vi "Create PMUs.vi"(8 "error in (no error)":errorcluster) -> (0 "error out":errorcluster)   [LabVIEW 2013, in "PMU Recorder Light.lvlib" / "Phasor Measurement Unit.lvclass"]
uses:
  Phasor Measurement Unit.lvclass
panel:
  in  "PMU Configuration":T1
  in  "Test Configuration":T1={"PMU Configuration"=[{"PMU ID Code"=3, "Station Name"="Hasle           ", "Nominal Frequency"=50.0, "Format Code"=8, "Configuration Change Count"=0, "Number of Phasors"=6, "Number of Analog"=0, "Number of Digital"=0, "Status"=TRUE}, {"PMU ID Code"=0, "Station Name"="NedreRossaga    ", "Nominal Frequency"=50.0, "Format Code"=8, "Configuration Change Count"=1, "Number of Phasors"=2, "Number of Analog"=0, "Number of Digital"=0, "Status"=TRUE}, {"PMU ID Code"=0, "Station Name"="Ben 667         ", "Nominal Frequency"=50.0, "Format Code"=8, "Configuration Change Count"=1, "Number of Phasors"=12, "Number of Analog"=0, "Number of Digital"=0, "Status"=TRUE}, {"PMU ID Code"=102, "Station Name"="Keminmaa        ", "Nominal Frequency"=50.0, "Format Code"=8, "Configuration Change Count"=4, "Number of Phasors"=6, "Number of Analog"=0, "Number of Digital"=0, "Status"=TRUE}, {"PMU ID Code"=113, "Station Name"="PETAJASKOSKI    ", "Nominal Frequency"=50.0, "Format Code"=8, "Configuration Change Count"=9, "Number of Phasors"=3, "Number of Analog"=0, "Number of Digital"=0, "Status"=TRUE}], "Phasor Configuration"=[{"Group Name"="Hasle", "Channel Name"="Halden-U", "Channel Name Real"="Halden-U", "Channel Name Imaginary"="Halden-U", "Group Index"=0, "Channel Index"=0, "isValid?"=TRUE, "Scaling"=20.97388, "Type"=0}, {"Group Name"="Hasle", "Channel Name"="Borgvik-U", "Channel Name Real"="Borgvik-U", "Channel Name Imaginary"="Borgvik-U", "Group Index"=0, "Channel Index"=1, "isValid?"=TRUE, "Scaling"=20.97388, "Type"=0}, {"Group Name"="Hasle", "Channel Name"="Borgvik-I", "Channel Name Real"="Borgvik-I", "Channel Name Imaginary"="Borgvik-I", "Group Index"=0, "Channel Index"=2, "isValid?"=TRUE, "Scaling"=0.54931, "Type"=1}, {"Group Name"="Hasle", "Channel Name"="Halden-I", "Channel Name Real"="Halden-I", "Channel Name Imaginary"="Halden-I", "Group Index"=0, "Channel Index"=3, "isValid?"=TRUE, "Scaling"=0.54931, "Type"=1}, {"Group Name"="Hasle", "Channel Name"="Roed-I", "Channel Name Real"="Roed-I", "Channel Name Imaginary"="Roed-I", "Group Index"=0, "Channel Index"=4, "isValid?"=TRUE, "Scaling"=0.54931, "Type"=1}, {"Group Name"="Hasle", "Channel Name"="Tegneby-I", "Channel Name Real"="Tegneby-I", "Channel Name Imaginary"="Tegneby-I", "Group Index"=0, "Channel Index"=5, "isValid?"=TRUE, "Scaling"=0.73242, "Type"=1}, {"Group Name"="NedreRossaga", "Channel Name"="Rana-U", "Channel Name Real"="Rana-U", "Channel Name Imaginary"="Rana-U", "Group Index"=1, "Channel Index"=0, "isValid?"=TRUE, "Scaling"=19.97513, "Type"=0}, {"Group Name"="NedreRossaga", "Channel Name"="Rana-I", "Channel Name Real"="Rana-I", "Channel Name Imaginary"="Rana-I", "Group Index"=1, "Channel Index"=1, "isValid?"=TRUE, "Scaling"=0.05493, "Type"=1}, {"Group Name"="Ben 667", "Channel Name"="420:Ba1:U_L1", "Channel Name Real"="420:Ba1:U_L1", "Channel Name Imaginary"="420:Ba1:U_L1", "Group Index"=2, "Channel Index"=0, "isValid?"=TRUE, "Scaling"=14.76031, "Type"=0}, {"Group Name"="Ben 667", "Channel Name"="420:Ba1:U_L2", "Channel Name Real"="420:Ba1:U_L2", "Channel Name Imaginary"="420:Ba1:U_L2", "Group Index"=2, "Channel Index"=1, "isValid?"=TRUE, "Scaling"=14.76031, "Type"=0}, {"Group Name"="Ben 667", "Channel Name"="420:Ba1:U_L3", "Channel Name Real"="420:Ba1:U_L3", "Channel Name Imaginary"="420:Ba1:U_L3", "Group Index"=2, "Channel Index"=2, "isValid?"=TRUE, "Scaling"=14.76031, "Type"=0}, {"Group Name"="Ben 667", "Channel Name"="420:Ba1:I_L1", "Channel Name Real"="420:Ba1:I_L1", "Channel Name Imaginary"="420:Ba1:I_L1", "Group Index"=2, "Channel Index"=3, "isValid?"=TRUE, "Scaling"=0.31169, "Type"=1}, {"Group Name"="Ben 667", "Channel Name"="420:Ba1:I_L2", "Channel Name Real"="420:Ba1:I_L2", "Channel Name Imaginary"="420:Ba1:I_L2", "Group Index"=2, "Channel Index"=4, "isValid?"=TRUE, "Scaling"=0.31169, "Type"=1}, {"Group Name"="Ben 667", "Channel Name"="420:Ba1:I_L3", "Channel Name Real"="420:Ba1:I_L3", "Channel Name Imaginary"="420:Ba1:I_L3", "Group Index"=2, "Channel Index"=5, "isValid?"=TRUE, "Scaling"=0.31169, "Type"=1}, {"Group Name"="Ben 667", "Channel Name"="420:Of1:U_L1", "Channel Name Real"="420:Of1:U_L1", "Channel Name Imaginary"="420:Of1:U_L1", "Group Index"=2, "Channel Index"=6, "isValid?"=TRUE, "Scaling"=14.76031, "Type"=0}, {"Group Name"="Ben 667", "Channel Name"="420:Of1:U_L2", "Channel Name Real"="420:Of1:U_L2", "Channel Name Imaginary"="420:Of1:U_L2", "Group Index"=2, "Channel Index"=7, "isValid?"=TRUE, "Scaling"=14.76031, "Type"=0}, {"Group Name"="Ben 667", "Channel Name"="420:Of1:U_L3", "Channel Name Real"="420:Of1:U_L3", "Channel Name Imaginary"="420:Of1:U_L3", "Group Index"=2, "Channel Index"=8, "isValid?"=TRUE, "Scaling"=14.76031, "Type"=0}, {"Group Name"="Ben 667", "Channel Name"="420:Of1:I_L1", "Channel Name Real"="420:Of1:I_L1", "Channel Name Imaginary"="420:Of1:I_L1", "Group Index"=2, "Channel Index"=9, "isValid?"=TRUE, "Scaling"=0.31169, "Type"=1}, {"Group Name"="Ben 667", "Channel Name"="420:Of1:I_L2", "Channel Name Real"="420:Of1:I_L2", "Channel Name Imaginary"="420:Of1:I_L2", "Group Index"=2, "Channel Index"=10, "isValid?"=TRUE, "Scaling"=0.31169, "Type"=1}, {"Group Name"="Ben 667", "Channel Name"="420:Of1:I_L3", "Channel Name Real"="420:Of1:I_L3", "Channel Name Imaginary"="420:Of1:I_L3", "Group Index"=2, "Channel Index"=11, "isValid?"=TRUE, "Scaling"=0.31169, "Type"=1}, {"Group Name"="Keminmaa", "Channel Name"="PK1", "Channel Name Real"="PK1", "Channel Name Imaginary"="PK1", "Group Index"=3, "Channel Index"=0, "isValid?"=TRUE, "Scaling"=21.97265, "Type"=0}, {"Group Name"="Keminmaa", "Channel Name"="PK2", "Channel Name Real"="PK2", "Channel Name Imaginary"="PK2", "Group Index"=3, "Channel Index"=1, "isValid?"=TRUE, "Scaling"=21.97265, "Type"=0}, {"Group Name"="Keminmaa", "Channel Name"="SELLEE 1.1/2", "Channel Name Real"="SELLEE 1.1/2", "Channel Name Imaginary"="SELLEE 1.1/2", "Group Index"=3, "Channel Index"=2, "isValid?"=TRUE, "Scaling"=0.27465, "Type"=1}, {"Group Name"="Keminmaa", "Channel Name"="SB 1.7/8", "Channel Name Real"="SB 1.7/8", "Channel Name Imaginary"="SB 1.7/8", "Group Index"=3, "Channel Index"=3, "isValid?"=TRUE, "Scaling"=0.54931, "Type"=1}, {"Group Name"="Keminmaa", "Channel Name"="PR 1.9/10", "Channel Name Real"="PR 1.9/10", "Channel Name Imaginary"="PR 1.9/10", "Group Index"=3, "Channel Index"=4, "isValid?"=TRUE, "Scaling"=0.27465, "Type"=1}, {"Group Name"="Keminmaa", "Channel Name"="PT 1.11/12", "Channel Name Real"="PT 1.11/12", "Channel Name Imaginary"="PT 1.11/12", "Group Index"=3, "Channel Index"=5, "isValid?"=TRUE, "Scaling"=0.54931, "Type"=1}, {"Group Name"="PETAJASKOSKI", "Channel Name"="V1LPM", "Channel Name Real"="V1LPM", "Channel Name Imaginary"="V1LPM", "Group Index"=4, "Channel Index"=0, "isValid?"=TRUE, "Scaling"=18.31055, "Type"=0}, {"Group Name"="PETAJASKOSKI", "Channel Name"="I1WPM", "Channel Name Real"="I1WPM", "Channel Name Imaginary"="I1WPM", "Group Index"=4, "Channel Index"=1, "isValid?"=TRUE, "Scaling"=0.32043, "Type"=1}, {"Group Name"="PETAJASKOSKI", "Channel Name"="I1XPM", "Channel Name Real"="I1XPM", "Channel Name Imaginary"="I1XPM", "Group Index"=4, "Channel Index"=2, "isValid?"=TRUE, "Scaling"=0.64087, "Type"=1}], "Analog Configuration"=[{"Group Name"="Hasle", "Channel Name"="frequency", "Group Index"=0, "Channel Index"=0, "isValid?"=TRUE, "Scaling"=1.0, "Type"=100}, {"Group Name"="Hasle", "Channel Name"="frequency-delta", "Group Index"=0, "Channel Index"=1, "isValid?"=TRUE, "Scaling"=1.0, "Type"=101}, {"Group Name"="NedreRossaga", "Channel Name"="frequency", "Group Index"=1, "Channel Index"=0, "isValid?"=TRUE, "Scaling"=1.0, "Type"=100}, {"Group Name"="NedreRossaga", "Channel Name"="frequency-delta", "Group Index"=1, "Channel Index"=1, "isValid?"=TRUE, "Scaling"=1.0, "Type"=101}, {"Group Name"="Ben 667", "Channel Name"="frequency", "Group Index"=2, "Channel Index"=0, "isValid?"=TRUE, "Scaling"=1.0, "Type"=100}, {"Group Name"="Ben 667", "Channel Name"="frequency-delta", "Group Index"=2, "Channel Index"=1, "isValid?"=TRUE, "Scaling"=1.0, "Type"=101}, {"Group Name"="Keminmaa", "Channel Name"="frequency", "Group Index"=3, "Channel Index"=0, "isValid?"=TRUE, "Scaling"=1.0, "Type"=100}, {"Group Name"="Keminmaa", "Channel Name"="frequency-delta", "Group Index"=3, "Channel Index"=1, "isValid?"=TRUE, "Scaling"=1.0, "Type"=101}, {"Group Name"="PETAJASKOSKI", "Channel Name"="frequency", "Group Index"=4, "Channel Index"=0, "isValid?"=TRUE, "Scaling"=1.0, "Type"=100}, {"Group Name"="PETAJASKOSKI", "Channel Name"="frequency-delta", "Group Index"=4, "Channel Index"=1, "isValid?"=TRUE, "Scaling"=1.0, "Type"=101}], "Digital Configuration"=[]}
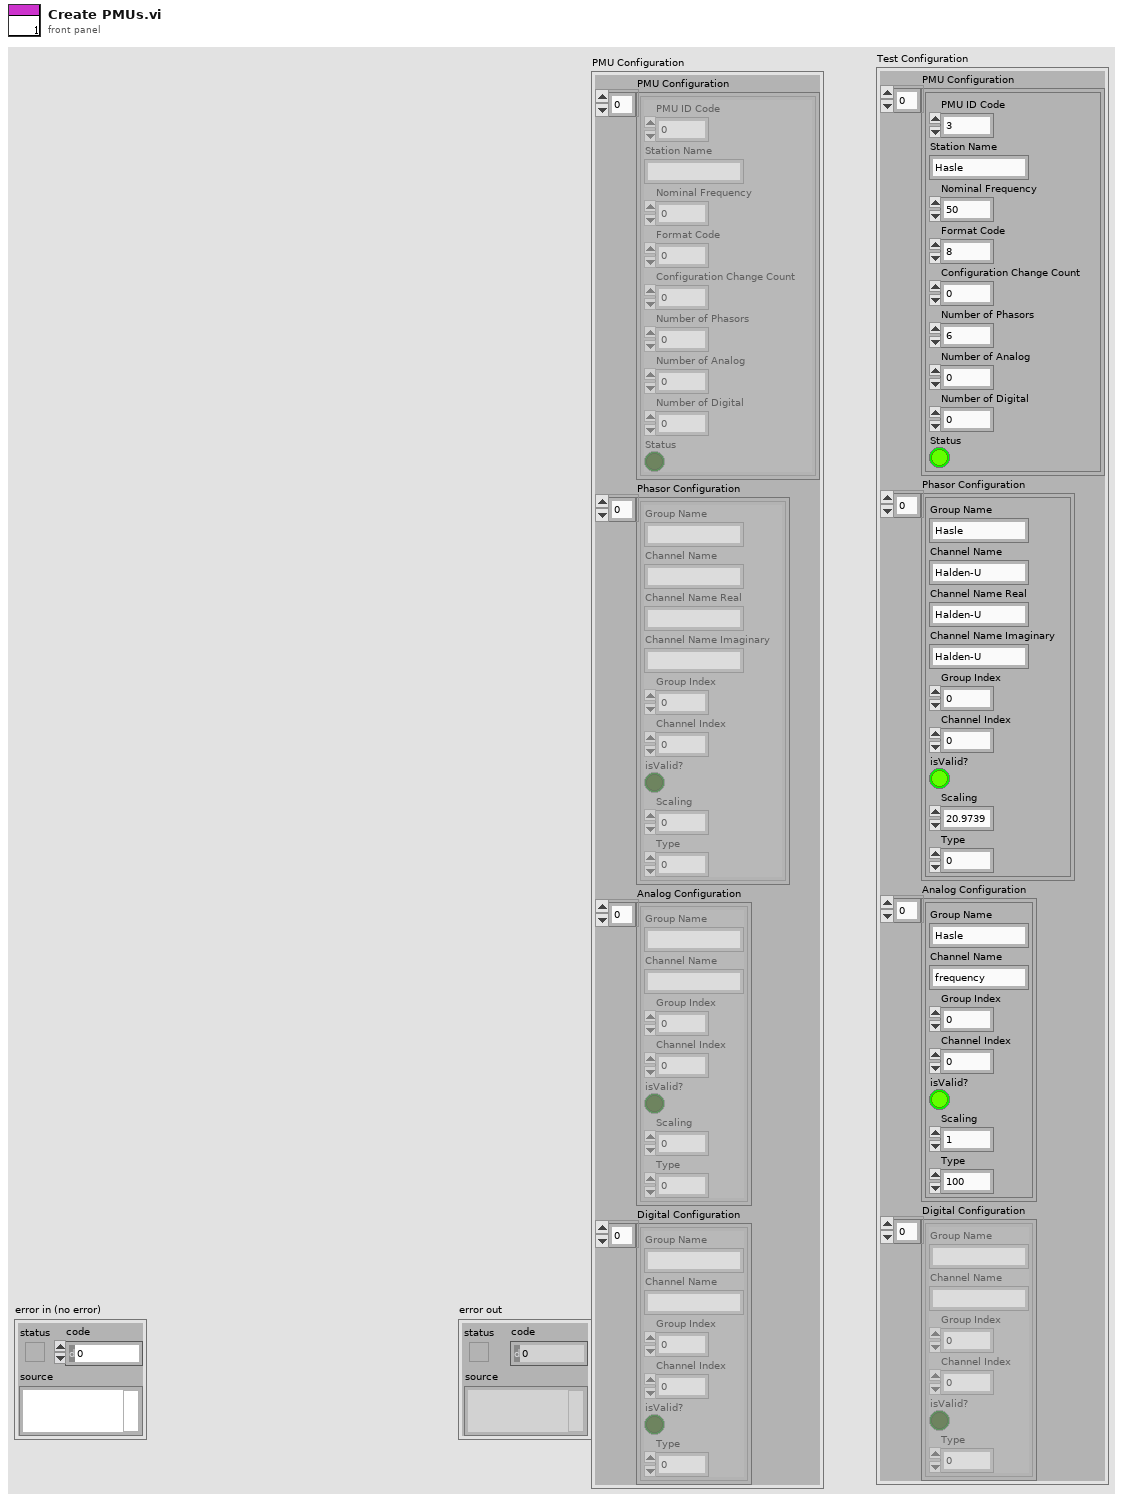
[diagram p1: front panel]
types:
  T1 = cluster{"PMU Configuration":cluster{"PMU ID Code":i32, "Station Name":string, "Nominal Frequency":sgl, "Format Code":i32, "Configuration Change Count":i32, "Number of Phasors":i32, "Number of Analog":i32, "Number of Digital":i32, "Status":bool}[], "Phasor Configuration":cluster{"Group Name":string, "Channel Name":string, "Channel Name Real":string, "Channel Name Imaginary":string, "Group Index":i32, "Channel Index":i32, "isValid?":bool, "Scaling":sgl, "Type":i32}[], "Analog Configuration":cluster{"Group Name":string, "Channel Name":string, "Group Index":i32, "Channel Index":i32, "isValid?":bool, "Scaling":sgl, "Type":i32}[], "Digital Configuration":cluster{"Group Name":string, "Channel Name":string, "Group Index":i32, "Channel Index":i32, "isValid?":bool, "Type":i32}[]}
  T2 = cluster{"PMU ID Code":i32, "Station Name":string, "Nominal Frequency":sgl, "Format Code":i32, "Configuration Change Count":i32, "Number of Phasors":i32, "Number of Analog":i32, "Number of Digital":i32, "Status":bool}[]
  T3 = cluster{"Group Name":string, "Channel Name":string, "Channel Name Real":string, "Channel Name Imaginary":string, "Group Index":i32, "Channel Index":i32, "isValid?":bool, "Scaling":sgl, "Type":i32}[]
  T4 = cluster{"Group Name":string, "Channel Name":string, "Group Index":i32, "Channel Index":i32, "isValid?":bool, "Scaling":sgl, "Type":i32}[]
  T5 = cluster{"Group Name":string, "Channel Name":string, "Group Index":i32, "Channel Index":i32, "isValid?":bool, "Type":i32}[]
  T6 = cluster{"Group Name":string, "Channel Name":string, "Channel Name Real":string, "Channel Name Imaginary":string, "Group Index":i32, "Channel Index":i32, "isValid?":bool, "Scaling":sgl, "Type":i32}
  T7 = cluster{"Group Name":string, "Channel Name":string, "Group Index":i32, "Channel Index":i32, "isValid?":bool, "Scaling":sgl, "Type":i32}
  T8 = cluster{"Group Name":string, "Channel Name":string, "Group Index":i32, "Channel Index":i32, "isValid?":bool, "Type":i32}
  T9 = cluster{"Cluster":cluster{"PMU ID Code":i32, "Station Name":string, "Nominal Frequency":sgl, "Format Code":i32, "Configuration Change Count":i32, "Number of Phasors":i32, "Number of Analog":i32, "Number of Digital":i32, "Status":bool}, cluster{"Group Name":string, "Channel Name":string, "Channel Name Real":string, "Channel Name Imaginary":string, "Group Index":i32, "Channel Index":i32, "isValid?":bool, "Scaling":sgl, "Type":i32}[], cluster{"Group Name":string, "Channel Name":string, "Group Index":i32, "Channel Index":i32, "isValid?":bool, "Scaling":sgl, "Type":i32}[], cluster{"Group Name":string, "Channel Name":string, "Group Index":i32, "Channel Index":i32, "isValid?":bool, "Type":i32}[]}
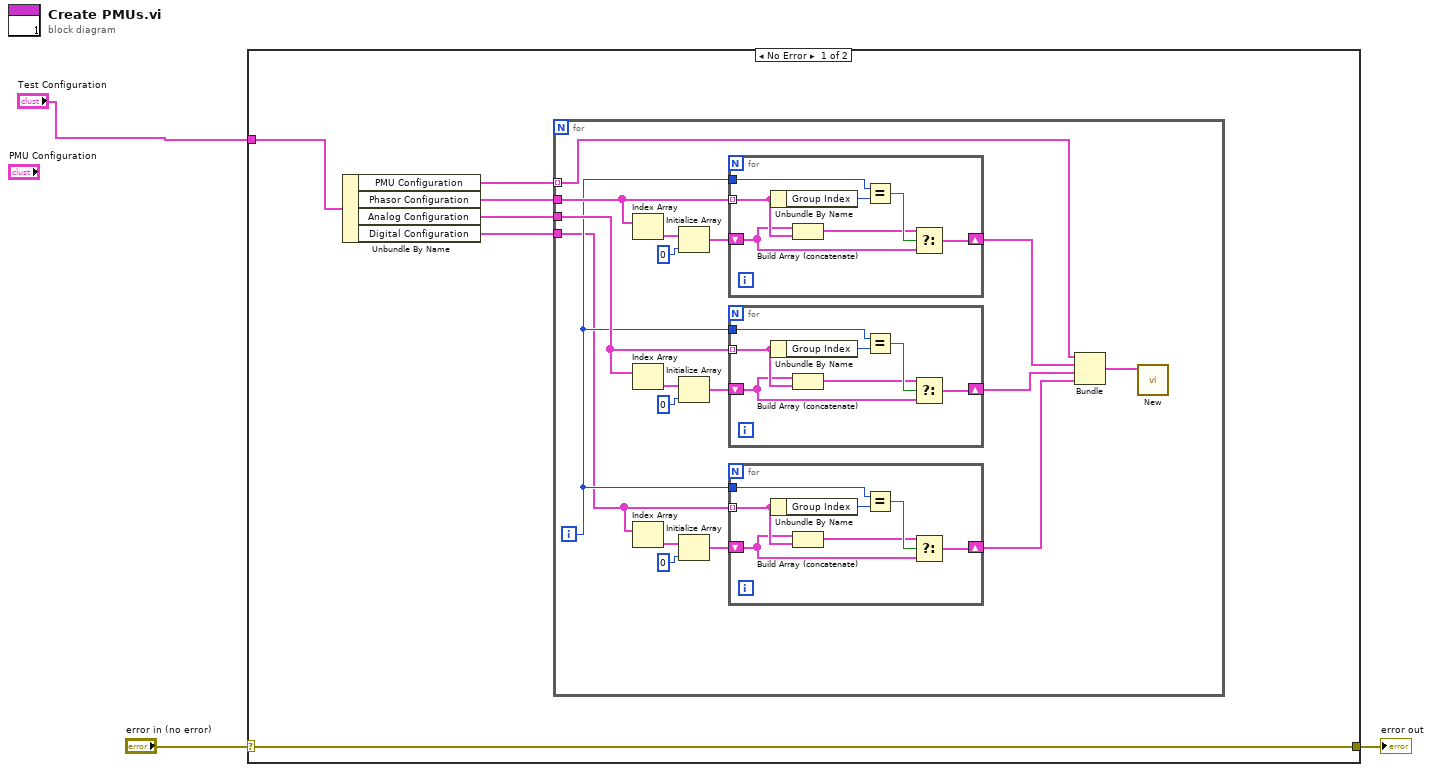
[diagram p0: block diagram]
diagram:
  n1 = case shown="No Error" "error in (no error)" {
    selector: "error in (no error)" -> [w9 w49]
    tunnel: [w9 w49] -> w2
    tunnel: "Test Configuration" -> [w8 _]
    frame No Error {
      n2 = Unbundle By Name(w8) -> ("PMU Configuration"=w7:T2, "Phasor Configuration"=w6:T3, "Analog Configuration"=w5:T4, "Digital Configuration"=w4:T5)
      n3 = for {
        tunnel: w7 -> [w11] mode=indexing
        tunnel: w6 -> [w27]
        tunnel: w5 -> [w20]
        tunnel: w4 -> [w15]
        i -> [w16]
        n4 = Index Array(array=w27) -> (element=w26:T6)  [unwired: 1 in]
        n5 = Index Array(array=w20) -> (element=w21:T7)  [unwired: 1 in]
        n6 = Index Array(array=w15) -> (element=w19:T8)  [unwired: 1 in]
        n7 = Initialize Array(w26, 0 ("dimension size")) -> (w24:T3)
        n8 = Initialize Array(w21, 0 ("dimension size")) -> (w23:T4)
        n9 = Initialize Array(w19, 0 ("dimension size")) -> (w17:T5)
        n10 = for {
          tunnel: w27 -> [w46] mode=indexing
          shift-right: [w44] -> w12
          shift-left: w24 -> [w42]
          tunnel: w16 -> [w47]
          n11 = Unbundle By Name(w46) -> ("Group Index"=w48:i32)
          n12 = Build Array (concatenate)(w42, w46) -> (w43:T3)
          n13 = Equal?(x=w47, y=w48) -> (x = y?=w45:bool)
          n14 = Select(t=w43, s=w45, f=w42) -> (s? t:f=w44:T3)
        }
        n15 = for {
          tunnel: w20 -> [w39] mode=indexing
          shift-right: [w37] -> w13
          shift-left: w23 -> [w35]
          tunnel: w16 -> [w40]
          n16 = Unbundle By Name(w39) -> ("Group Index"=w41:i32)
          n17 = Build Array (concatenate)(w35, w39) -> (w36:T4)
          n18 = Equal?(x=w40, y=w41) -> (x = y?=w38:bool)
          n19 = Select(t=w36, s=w38, f=w35) -> (s? t:f=w37:T4)
        }
        n20 = for {
          tunnel: w15 -> [w32] mode=indexing
          shift-right: [w30] -> w14
          shift-left: w17 -> [w28]
          tunnel: w16 -> [w33]
          n21 = Unbundle By Name(w32) -> ("Group Index"=w34:i32)
          n22 = Build Array (concatenate)(w28, w32) -> (w29:T5)
          n23 = Equal?(x=w33, y=w34) -> (x = y?=w31:bool)
          n24 = Select(t=w29, s=w31, f=w28) -> (s? t:f=w30:T5)
        }
        n25 = Bundle("Cluster"=w11, w12, w13, w14) -> (w10:T9)  [unwired: 1 in]
        n26 = call "New.vi"("PMU Configuration"=w10) -> ()  [unwired: 9 in, 2 out]
      }
    }
    frame Error {
    }
  }
  "error out" <- w2
